vi "Write plots.vi"(5 "plots":refnum<class "Plot.lvclass">[](array[class]), 9 "WaveformGraph in":refnum<class "WaveformGraph.lvclass">) -> (3 "WaveformGraph out":refnum<class "WaveformGraph.lvclass">)   [LabVIEW 2014, in "WaveformGraph.lvclass"]
uses:
  WaveformGraph.lvclass
  Plot/Plot.lvclass
  WaveformGraph.lvclass/WaveformGraph.ctl
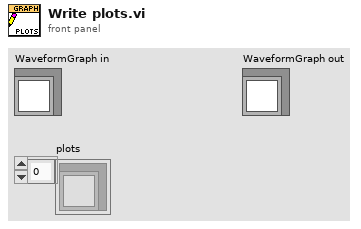
[diagram p1: front panel]
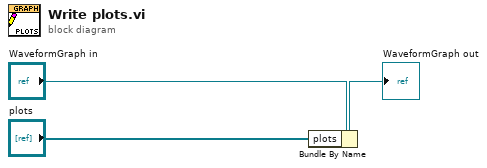
[diagram p0: block diagram]
diagram:
  n1 = Bundle By Name(cluster="WaveformGraph in", "plots"="plots") -> (→"WaveformGraph out":refnum<class "WaveformGraph.lvclass">)
